vi "DAQ_Mic.vi"() -> ()   [LabVIEW 2020]
panel:
  in  "stop":bool
  out "Waveform Graph":dynamicdata(graph)
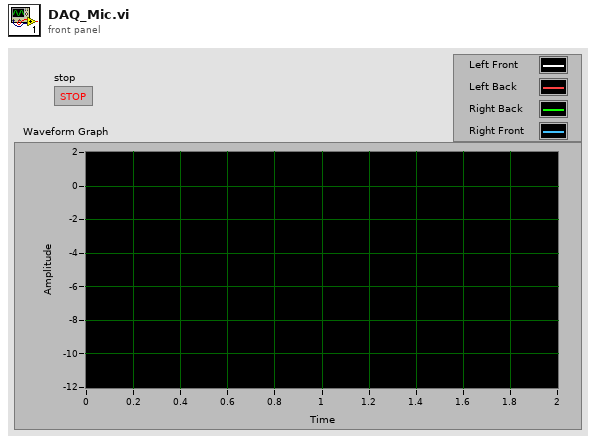
[diagram p1: front panel]
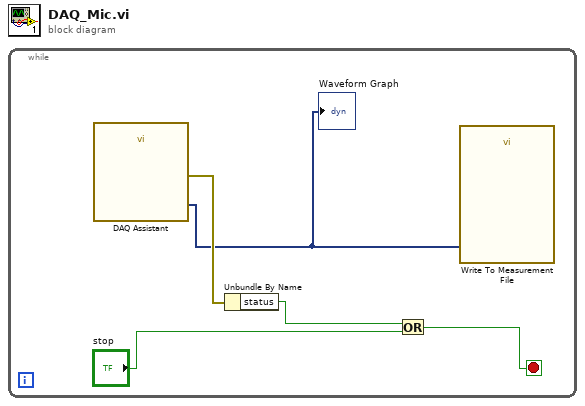
[diagram p0: block diagram]
diagram:
  n1 = while {
    stop <- w1 stop-if-true
    n2 = call "DAQ Assistant"() -> ("data"=w3:dynamicdata, "error out"=w4:errorcluster)  [unwired: 17 in, 1 out]
    "Waveform Graph" <- w3
    n3 = Unbundle By Name(w4) -> ("status"=w5:bool)
    n4 = Or(x=w5, y="stop") -> (x .or. y?=w1:bool)
    n5 = call "Write To Measurement File"("Signals"=w3) -> ()  [unwired: 16 in, 3 out]
  }
